vi "Read Axis BMP.vi"(8 "error in (no error) 2":errorcluster, 9 "CGI?":bool=TRUE, 10 "Acquire Params":T1={"fps"=10, "Compression"=30, "X"=320, "Y"=240, "Enable Color?"=TRUE, "Rotation"=enum."0"}, 11 "address":string="192.168.1.101") -> (0 "error out":errorcluster, 3 "Raw Image Data":string)   [LabVIEW 2017]
panel:
  out "concatenated string":string
  # "NEEDED: get image size from stream instead of 320x240 constant.\nHandle HTTP errors\nReverse rows, not entire array, currently HMirror.\nUse BuildCGI subVI"
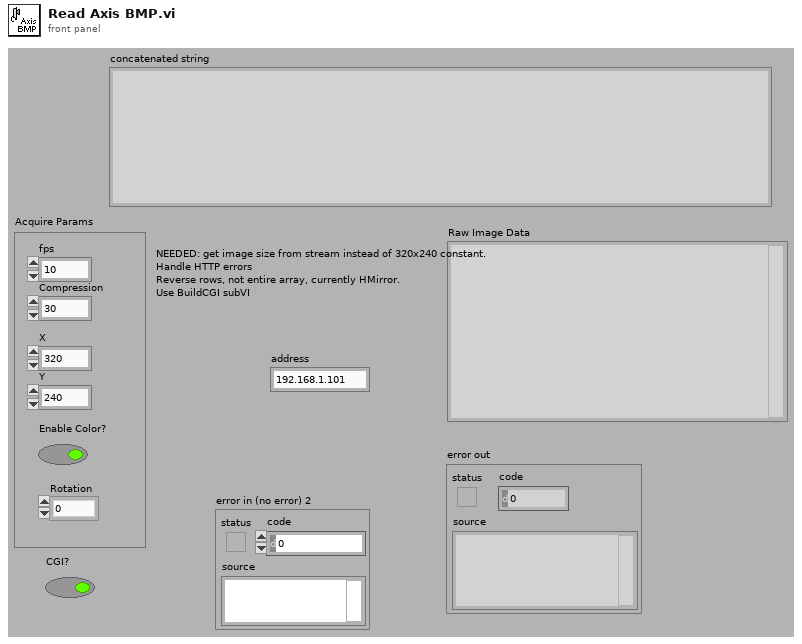
[diagram p1: front panel]
types:
  T1 = cluster{"fps":i32, "Compression":i32, "X":i32, "Y":i32, "Enable Color?":bool, "Rotation":enum16{"0", "90", "180", "270"}}
  T2 = enum16{"Standard", "Buffered", "CRLF", "Immediate"}
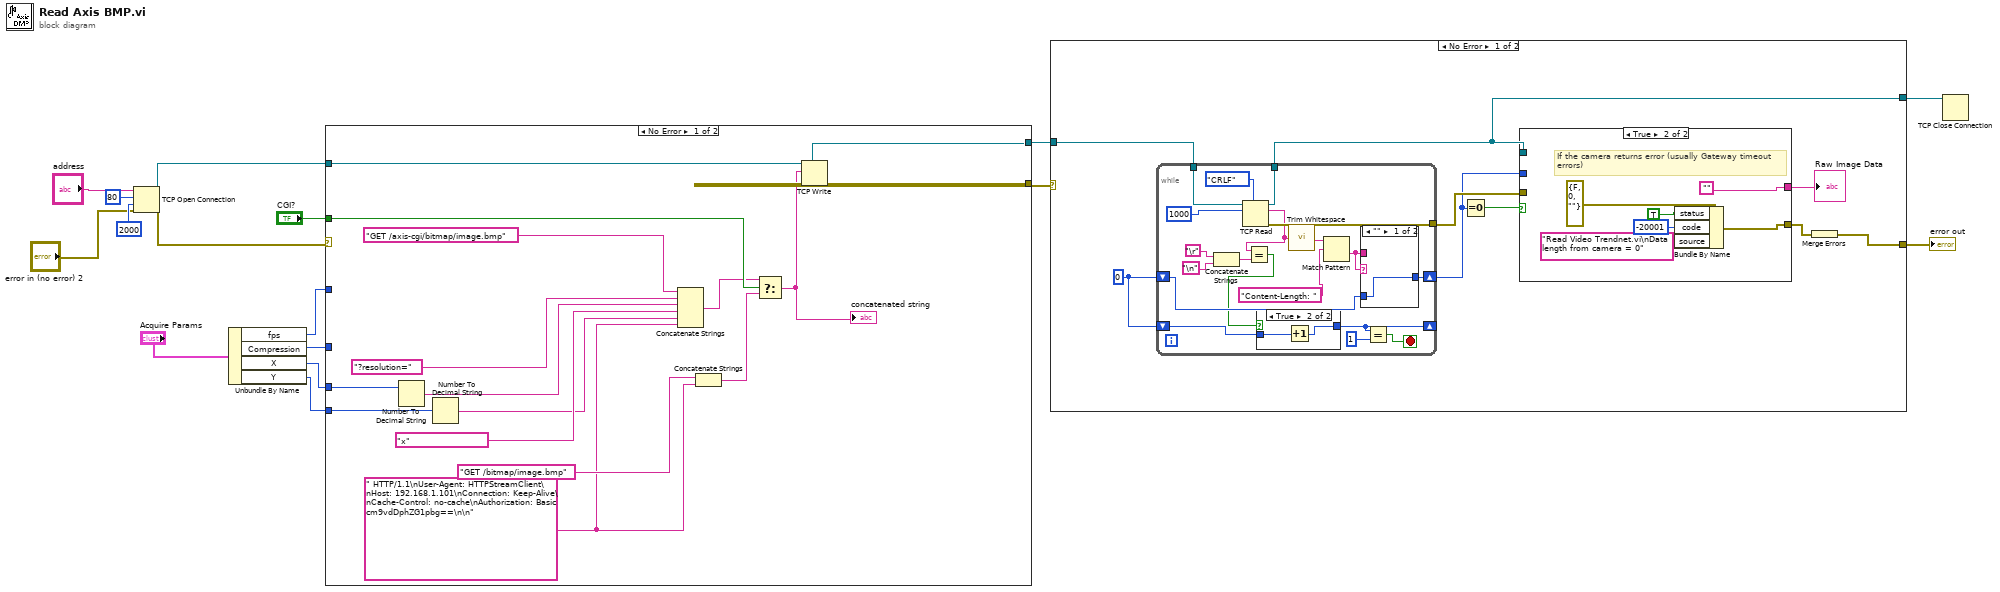
[diagram p0: block diagram]
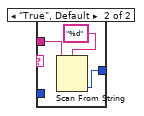
[diagram p3: hidden frame]
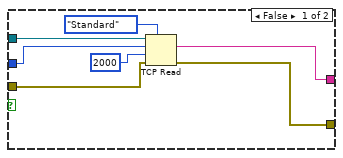
[diagram p4: hidden frame]
diagram:
  n1 = TCP Open Connection(address="address", remote port or service name=u16 80, timeout ms (60000)=2000, error in (no error)="error in (no error) 2") -> (connection ID=w11:refnum<k5>, error out=w12:errorcluster)  [unwired: 1 in]
  n2 = Unbundle By Name("Acquire Params") -> ("fps"=w6:i32, "Compression"=w5:i32, "X"=w4:i32, "Y"=w3:i32)
  n3 = case shown="No Error" w12 {
    selector: w12 -> [_ w34]
    tunnel: [w32 w34] -> w8
    tunnel: w11 -> [w31 w33]
    tunnel: [w30 w33] -> w7
    tunnel: w6 -> [_ _]
    tunnel: w5 -> [_ _]
    tunnel: w4 -> [w25 _]
    tunnel: w3 -> [w24 _]
    tunnel: "CGI?" -> [w21 _]
    frame No Error {
      w18 = " HTTP/1.1\nUser-Agent: HTTPStreamClient\nHost: 192.168.1.101\nConnection: Keep-Alive\nCache-Control: no-cache\nAuthorization: Basic cm9vdDphZG1pbg==\n\n"
      n4 = Number To Decimal String(number=w25) -> (decimal integer string=w28:string)  [unwired: 1 in]
      n5 = Number To Decimal String(number=w24) -> (decimal integer string=w26:string)  [unwired: 1 in]
      n6 = Concatenate Strings("GET /axis-cgi/bitmap/image.bmp", "?resolution=", w28, "x", w26, w18) -> (w17:string)
      n7 = Concatenate Strings("GET /bitmap/image.bmp", w18) -> (w20:string)
      n8 = Select(t=w17, s=w21, f=w20) -> (s? t:f=w22:string)
      "concatenated string" <- w22
      n9 = TCP Write(connection ID=w31, data in=w22) -> (connection ID out=w30:refnum<k5>, error out=w32:errorcluster)  [unwired: 2 in, 1 out]
    }
    frame Error {
    }
  }
  n10 = case shown="No Error" w8 {
    selector: w8 -> [_ w84]
    tunnel: [w42 w84] -> w9
    tunnel: w7 -> [w37 w83]
    tunnel: [w35 w83] -> w2
    frame No Error {
      w36 = 0
      n11 = while {
        tunnel: w37 -> [w61]
        tunnel: [w59] -> w35
        tunnel: [w58] -> w39
        shift-right: [w51] -> w38
        shift-left: w36 -> [w50]
        shift-right: [w46] -> _
        shift-left: w36 -> [w48]
        stop <- w47 stop-if-true
        n12 = Concatenate Strings("\r", "\n") -> (w55:string)
        n13 = TCP Read(connection ID=w61, bytes to read=1000, 7:T2."CRLF" ("mode (standard)")) -> (connection ID out=w59:refnum<k5>, data out=w44:string, error out=w58:errorcluster)  [unwired: 2 in]
        n14 = Equal?(x=w44, y=w55) -> (x = y?=w49:bool)
        n15 = case shown="True" w49 {
          tunnel: w48 -> [w63 w65]
          tunnel: [w63 w64] -> w46
          frame False {
          }
          frame True {
            n16 = Increment(x=w65) -> (x+1=w64:i32)
          }
        }
        n17 = call <vilib>:"Trim Whitespace.vi"("string"=w44) -> ("trimmed string"=w53:string)  [unwired: 1 in]
        n18 = Match Pattern(string=w53, regular expression="Content-Length: ") -> (after substring=w52:string)  [unwired: 1 in, 3 out]
        n19 = case shown="\"\"" w52 {
          tunnel: w52 -> [_ w69]
          tunnel: [w66 w67] -> w51
          tunnel: w50 -> [w66 _]
          frame "" {
          }
          frame "True", Default {
            n20 = Scan From String(format string="%d", input string=w69) -> (output 1=w67:i32)  [unwired: 3 in, 3 out]
          }
        }
        n21 = Equal?(x=w46, y=1) -> (x = y?=w47:bool)
      }
      n22 = Equal To 0?(x=w38) -> (x = 0?=w40:bool)
      n23 = case shown="True" w40 {
        tunnel: w35 -> [w76 _]
        tunnel: w39 -> [w75 _]
        tunnel: [w74 w82] -> w43
        tunnel: [w70 ""] -> w41
        tunnel: w38 -> [w71 _]
        frame False {
          n24 = TCP Read(connection ID=w76, bytes to read=w71, error in (no error)=w75, 7:T2."Standard" ("mode (standard)"), 9:2000 ("timeout ms (25000)")) -> (data out=w70:string, error out=w74:errorcluster)  [unwired: 1 out]
        }
        frame True {
          # "If the camera returns error (usually Gateway timeout\nerrors)"
          n25 = Bundle By Name(cluster=errorcluster {"status"=FALSE, "code"=0, "source"=""} ("error in"), "status"=TRUE, "code"=-20001, "source"="Read Video Trendnet.vi\nData length from camera = 0") -> (w82:errorcluster)
        }
      }
      "Raw Image Data" <- w41
      n26 = Merge Errors(w43) -> (w42:errorcluster)
    }
    frame Error {
    }
  }
  "error out" <- w9
  n27 = TCP Close Connection(connection ID=w2) -> ()  [unwired: 2 in, 2 out]
